vi "String - Create Caption Paths.vi"(6 "LanguageID":string, 9 "name or relative path":string, 10 "Current VI's path":path, 11 "Path in":refnum<vi>) -> (2 "xml Path":path, 3 "VI Path":path)   [LabVIEW 2013]
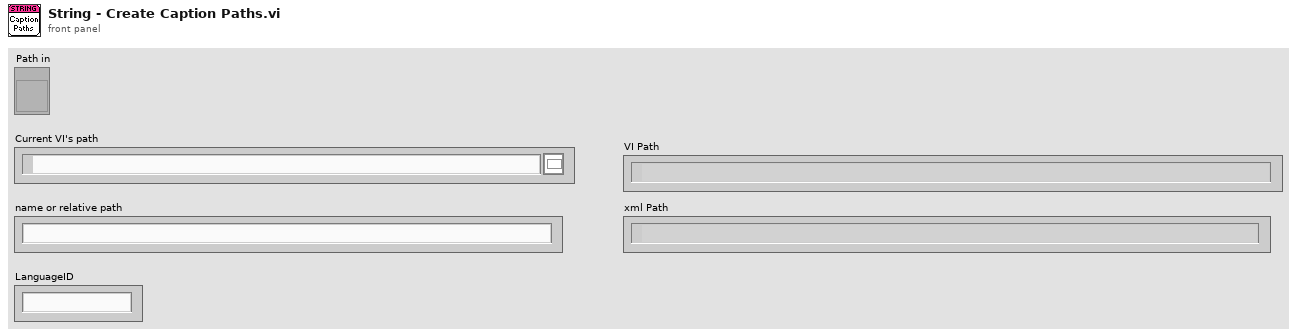
[diagram p1: front panel]
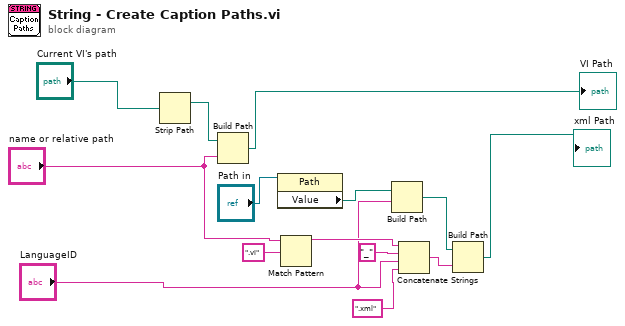
[diagram p0: block diagram]
diagram:
  n1 = Strip Path(path="Current VI's path") -> (stripped path=w4:path)  [unwired: 1 out]
  n2 = Build Path(base path=w4, name or relative path="name or relative path") -> (appended path=→"VI Path":path)
  n3 = property class="Path"(reference="Path in") -> ("Value"=w6:path)  [unwired: 1 in, 2 out]
  n4 = Match Pattern(string="name or relative path", regular expression=".vi") -> (before substring=w10:string)  [unwired: 1 in, 3 out]
  n5 = Build Path(base path=w6, name or relative path="LanguageID") -> (appended path=w12:path)
  n6 = Concatenate Strings(w10, "_" ("string"), "LanguageID", ".xml" ("string")) -> (w13:string)
  n7 = Build Path(base path=w12, name or relative path=w13) -> (appended path=→"xml Path":path)
